vi "DOCK_GEAR_get_operations_and_results.vi"(6 "executed_SQL_statement_in":string, 8 "error_in":errorcluster, 11 "SQL_result":variant) -> (0 "error_out":errorcluster, 2 "current_batch_ID":string, 3 "NOK_stations":string[](array[string]), 4 "executed_SQL_statement_out":string)   [LabVIEW 2019]
uses:
  FGV/DOCK_records_display/FGV_DOCK_records_display.ctl
  FGV/SQL_connection/FGV_DOCK_SQL_connection.ctl
  _misc/AULocalize/SubVIs/Get Localized Phrase Compact Interface 0D.vi
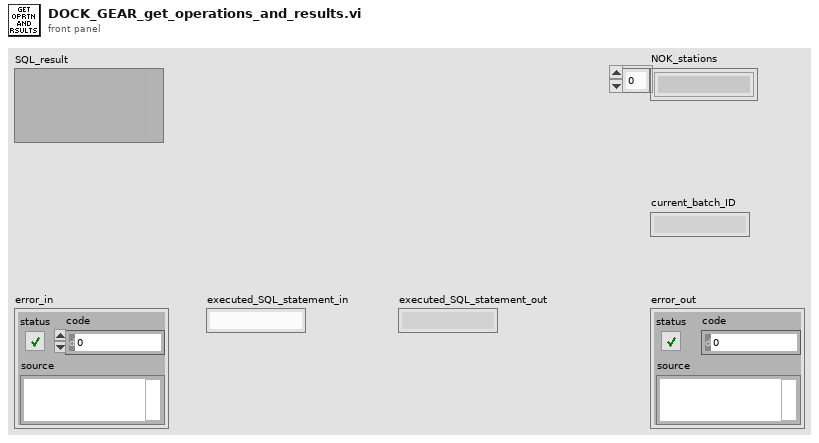
[diagram p1: front panel]
types:
  T1 = typedef "FGV_DOCK_records_display.ctl" = enum16{"initialize", "set_reference_data", "set_serial", "set_header", "set_operations", "set_results", "set_batches", "get_reference_data", "get_part_number_ref", "get_serial", "get_batch_code", "get_gear_ID", "get_operation_IDs", "toggle_results", "show_all_results", "hide_all_results", "display", "clear"}
  T2 = typedef "FGV_DOCK_SQL_connection.ctl" = enum16{"initialize", "connect", "read_tables", "read_columns", "SELECT", "INSERT", "UPDATE", "DELETE", "EXEC + headers", "EXEC", "TRANSACTION", "connection_active?", "disconnect"}
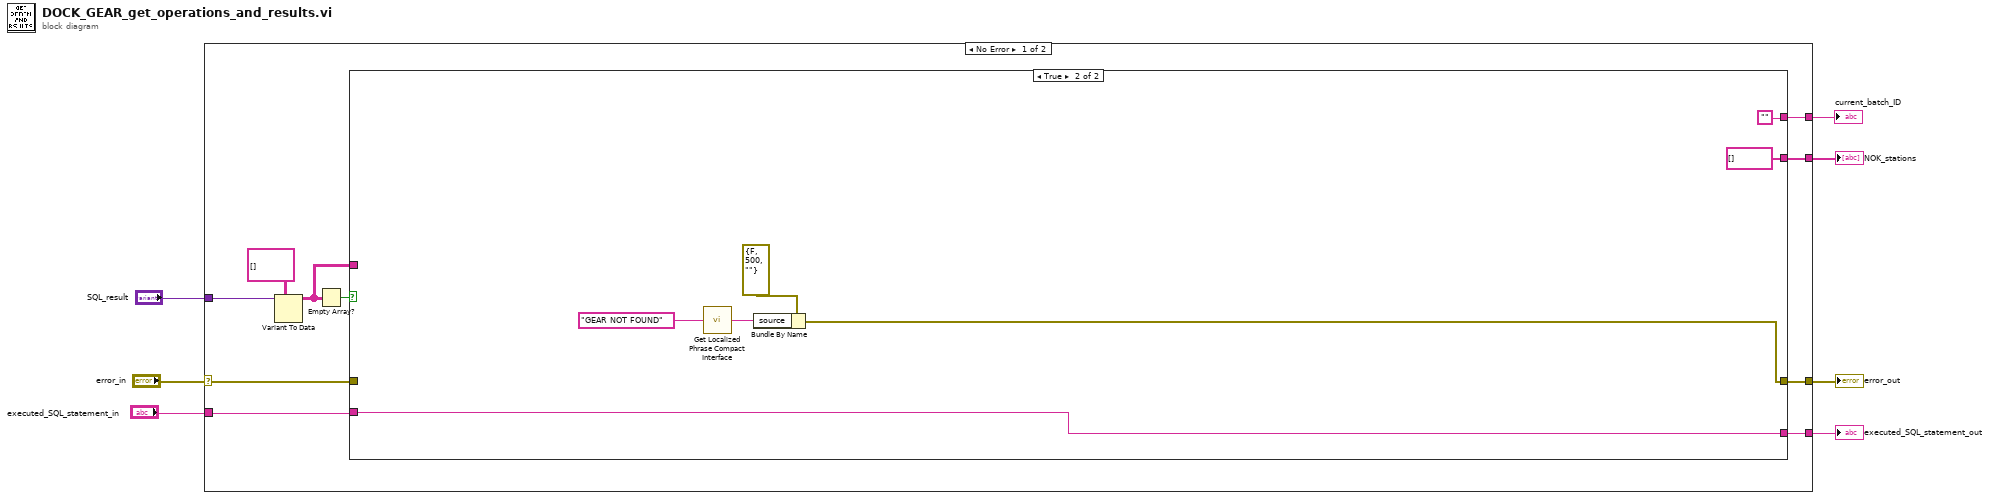
[diagram p0: block diagram]
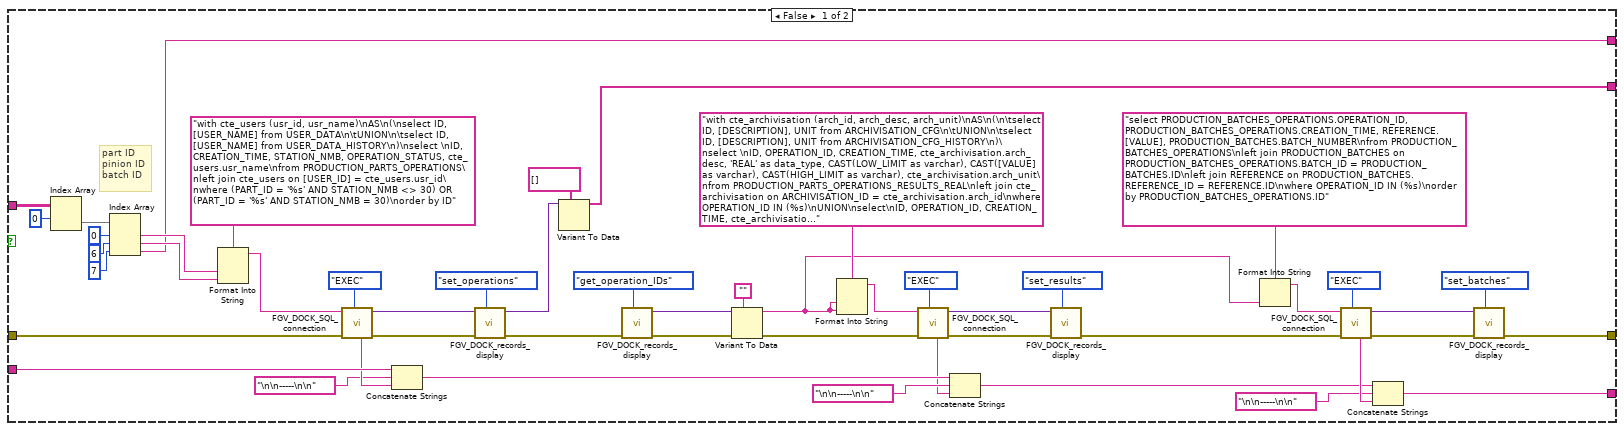
[diagram p2: hidden frame]
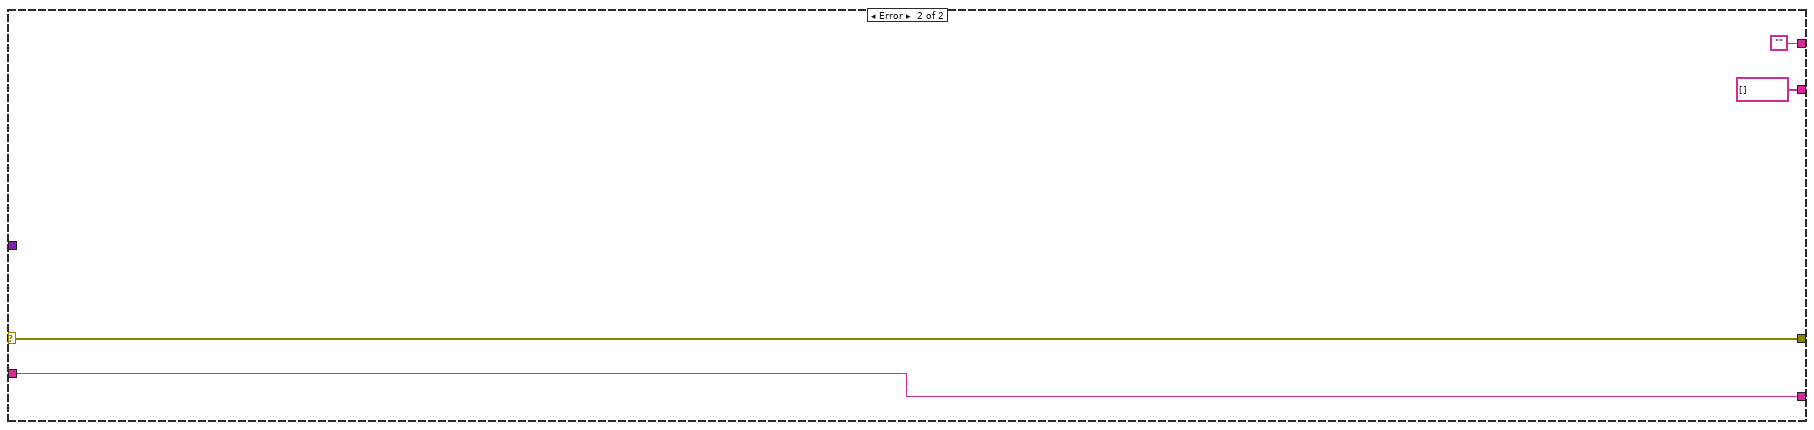
[diagram p3: hidden frame]
diagram:
  n1 = case shown="No Error" "error_in" {
    selector: "error_in" -> [w14 w78]
    tunnel: [w17 w77] -> w7
    tunnel: "executed_SQL_statement_in" -> [w16 w77]
    tunnel: [w15 w78] -> w5
    tunnel: "SQL_result" -> [w13 _]
    tunnel: [w9 string[] []] -> w2
    tunnel: [w8 ""] -> w1
    frame No Error {
      n2 = Variant To Data(type=string[][] [], Variant=w13) -> (data=w11:string[][])  [unwired: 1 in, 1 out]
      n3 = Empty Array?(array=w11) -> (empty?=w12:bool)
      n4 = case shown="True" w12 {
        tunnel: w14 -> [w67 _]
        tunnel: [w28 w70] -> w15
        tunnel: w16 -> [w53 w74]
        tunnel: [w26 w74] -> w17
        tunnel: w11 -> [w62 _]
        tunnel: [w20 string[] []] -> w9
        tunnel: [w18 ""] -> w8
        frame False {
          # "part ID\npinion ID\nbatch ID"
          n5 = Index Array(array=w62, index (row)=0) -> (element=w60:string[])  [unwired: 1 in]
          n6 = Index Array(array=w60, index #1=0 ("index"), index #2=6 ("index"), index #3=7 ("index")) -> (element #1=w55:string, element #2=w54:string, element #3=w18:string)
          n7 = Format Into String(format string="with cte_users (usr_id, usr_name)\nAS\n(\nselect ID, [USER_NAME] from USER_DATA\n\tUNION\n\tselect ID, [USER_NAME] from USER_DATA_HISTORY\n)\nselect \nID, CREATION_TIME, STATION_NMB, OPERATION_STATUS, cte_users.usr_name\nfrom PRODUCTION_PARTS_OPERATIONS\nleft join cte_users on [USER_ID] = cte_users.usr_id\nwhere (PART_ID = '%s' AND STATION_NMB <> 30) OR (PART_ID = '%s' AND STATION_NMB = 30)\norder by ID", w55, w54) -> (resulting string=w57:string)  [unwired: 2 in, 1 out]
          n8 = call "FGV_DOCK_SQL_connection.vi"("options"=FGV_DOCK_SQL_connection."EXEC", "error_in"=w67, "SQL_statement"=w57) -> ("error_out"=w64:errorcluster, "SQL_result"=w63:variant, "executed_SQL_statement"=w52:string)  [unwired: 4 in, 2 out]
          n9 = Concatenate Strings(w53, "\n\n-----\n\n" ("string"), w52) -> (w45:string)
          n10 = call "FGV_DOCK_records_display.vi"("options"=FGV_DOCK_records_display."set_operations", "error_in"=w64, "input"=w63) -> ("error_out"=w41:errorcluster, "output"=w22:variant)  [unwired: 7 in]
          n11 = Variant To Data(type=string[] [], Variant=w22) -> (data=w20:string[])  [unwired: 1 in, 1 out]
          n12 = call "FGV_DOCK_records_display.vi"("options"=FGV_DOCK_records_display."get_operation_IDs", "error_in"=w41) -> ("error_out"=w24:errorcluster, "output"=w39:variant)  [unwired: 8 in]
          n13 = Variant To Data(error in=w24, type="", Variant=w39) -> (data=w25:string, error out=w23:errorcluster)
          n14 = Format Into String(format string="with cte_archivisation (arch_id, arch_desc, arch_unit)\nAS\n(\n\tselect ID, [DESCRIPTION], UNIT from ARCHIVISATION_CFG\n\tUNION\n\tselect ID, [DESCRIPTION], UNIT from ARCHIVISATION_CFG_HISTORY\n)\nselect \nID, OPERATION_ID, CREATION_TIME, cte_archivisation.arch_desc, 'REAL' as data_type, CAST(LOW_LIMIT as varchar), CAST([VALUE] as varchar), CAST(HIGH_LIMIT as varchar), cte_archivisation.arch_unit\nfrom PRODUCTION_PARTS_OPERATIONS_RESULTS_REAL\nleft join cte_archivisation on ARCHIVISATION_ID = cte_archivisation.arch_id\nwhere OPERATION_ID IN (%s)\nUNION\nselect\nID, OPERATION_ID, CREATION_TIME, cte_archivisation.arch_desc, 'STRING' as data_type, '-', [VALUE], '-', cte_archivisation.arch_unit\nfrom PRODUCTION_PARTS_OPERATIONS_RESULTS_STRING\nleft join cte_archivisation on ARCHIVISATION_ID = cte_archivisation.arch_id\nwhere OPERATION_ID IN (%s)\norder by data_type, ID", w25, w25) -> (resulting string=w43:string)  [unwired: 2 in, 1 out]
          n15 = call "FGV_DOCK_SQL_connection.vi"("options"=FGV_DOCK_SQL_connection."EXEC", "error_in"=w23, "SQL_statement"=w43) -> ("error_out"=w48:errorcluster, "SQL_result"=w50:variant, "executed_SQL_statement"=w44:string)  [unwired: 4 in, 2 out]
          n16 = Concatenate Strings(w45, "\n\n-----\n\n" ("string"), w44) -> (w27:string)
          n17 = call "FGV_DOCK_records_display.vi"("options"=FGV_DOCK_records_display."set_results", "error_in"=w48, "input"=w50) -> ("error_out"=w29:errorcluster)  [unwired: 7 in, 1 out]
          n18 = Format Into String(format string="select PRODUCTION_BATCHES_OPERATIONS.OPERATION_ID, PRODUCTION_BATCHES_OPERATIONS.CREATION_TIME, REFERENCE.[VALUE], PRODUCTION_BATCHES.BATCH_NUMBER\nfrom PRODUCTION_BATCHES_OPERATIONS\nleft join PRODUCTION_BATCHES on PRODUCTION_BATCHES_OPERATIONS.BATCH_ID = PRODUCTION_BATCHES.ID\nleft join REFERENCE on PRODUCTION_BATCHES.REFERENCE_ID = REFERENCE.ID\nwhere OPERATION_ID IN (%s)\norder by PRODUCTION_BATCHES_OPERATIONS.ID", w25) -> (resulting string=w36:string)  [unwired: 2 in, 1 out]
          n19 = call "FGV_DOCK_SQL_connection.vi"("options"=FGV_DOCK_SQL_connection."EXEC", "error_in"=w29, "SQL_statement"=w36) -> ("error_out"=w32:errorcluster, "SQL_result"=w30:variant, "executed_SQL_statement"=w35:string)  [unwired: 4 in, 2 out]
          n20 = Concatenate Strings(w27, "\n\n-----\n\n" ("string"), w35) -> (w26:string)
          n21 = call "FGV_DOCK_records_display.vi"("options"=FGV_DOCK_records_display."set_batches", "error_in"=w32, "input"=w30) -> ("error_out"=w28:errorcluster)  [unwired: 7 in, 1 out]
        }
        frame True {
          n22 = call-poly "Get Localized Phrase Compact Interface.vi"("Key"="GEAR NOT FOUND" ("source")) -> ("Translated Phrase"=w68:string)
          n23 = Bundle By Name(cluster=errorcluster {"status"=FALSE, "code"=500, "source"=""} ("error IO"), "source"=w68) -> (w70:errorcluster)
        }
      }
    }
    frame Error {
    }
  }
  "executed_SQL_statement_out" <- w7
  "error_out" <- w5
  "NOK_stations" <- w2
  "current_batch_ID" <- w1
